vi "MERGE DAQ and DAQmx .Sampling.Configure.vi"(8 "error in (no error)":errorcluster, 11 "Instrument.DAQ":refnum<class "Instrument.DAQ.lvclass">) -> (0 "error out":errorcluster, 2 "Restart Acquisition?":bool, 3 "Instrument.DAQ out":refnum<class "Instrument.DAQ.lvclass">)   [LabVIEW 2019, in "Instrument.Lockin.lvlib" / "Instrument.DAQ.lvclass"]
uses:
  Instrument.DAQ.lvclass
  Instrument.DAQ.lvclass/Instrument.DAQ.ctl
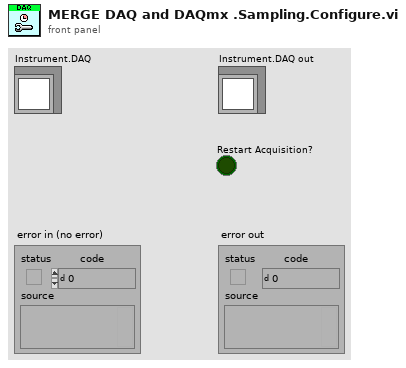
[diagram p1: front panel]
types:
  T1 = typedef "Instrument.Lockin.lvlib/Instrument.DAQ.lvclass/DAQ.Sampling--Cluster.ctl" = cluster{"Sampling":T2, "Fs_Out":dbl}
  T2 = typedef "Instrument.Lockin.lvlib/Instrument.DAQ.lvclass/DAQ.Sampling.Sampling--Cluster.ctl" = cluster{"Fs":dbl, "#s":i32}
  T3 = cluster{"Sampling":cluster{"Fs":bool, "#s":bool}, "Fs_Out":bool}
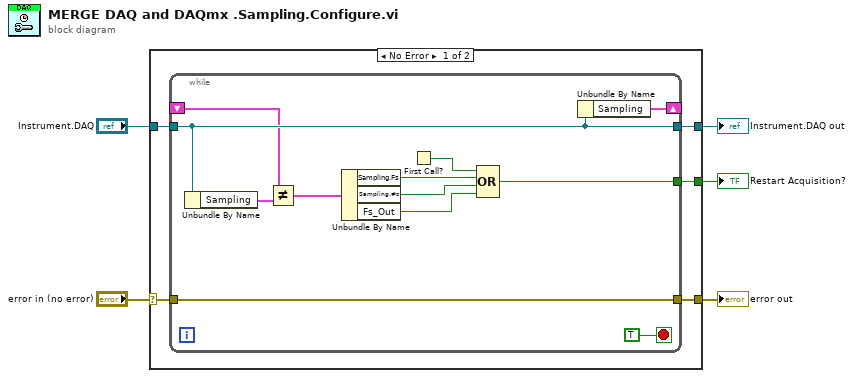
[diagram p0: block diagram]
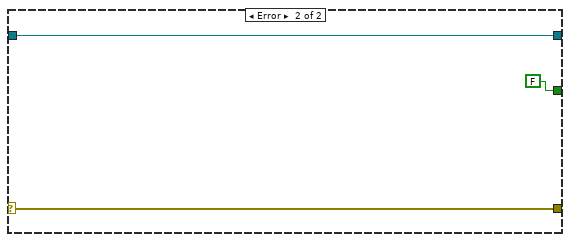
[diagram p2: hidden frame]
diagram:
  n1 = case shown="No Error" "error in (no error)" {
    selector: "error in (no error)" -> [w9 w25]
    tunnel: "Instrument.DAQ" -> [w10 w24]
    tunnel: [w6 w24] -> w3
    tunnel: [w8 w25] -> w2
    tunnel: [w7 FALSE] -> w1
    frame No Error {
      n2 = while {
        tunnel: [w13] -> w7
        tunnel: w10 -> [w19]
        tunnel: [w19] -> w6
        tunnel: w9 -> [w20]
        tunnel: [w20] -> w8
        shift-right: [w21] -> _
        shift-left: _ -> [w11]
        stop <- TRUE stop-if-true
        n3 = Unbundle By Name(w19) -> ("Sampling"=w12:T1)
        n4 = Not Equal?(x=w11, y=w12) -> (x != y?=w14:T3)
        n5 = Unbundle By Name(w14) -> ("Sampling.Fs"=w18:bool, "Sampling.#s"=w17:bool, "Fs_Out"=w16:bool)
        n6 = First Call?() -> (First Call?: T/F=w15:bool)
        n7 = Compound Arithmetic op=OR(w15, w18, w17, w16) -> (w13:bool)
        n8 = Unbundle By Name(w19) -> ("Sampling"=w21:T1)
      }
    }
    frame Error {
    }
  }
  "Instrument.DAQ out" <- w3
  "error out" <- w2
  "Restart Acquisition?" <- w1
